vi "inputRead.vi"() -> (10 "ADIO":bool[](array[boolean]), 11 "BDI1":bool[](array[boolean]), 12 "ADI1":bool[](array[boolean]), 13 "BDI0":bool[](array[boolean]), 14 "ADI2":bool[](array[boolean]), 15 "ADI15":bool[](array[boolean]), 16 "ADI3":bool[](array[boolean]), 17 "ADI14":bool[](array[boolean]), 18 "ADI4":bool[](array[boolean]), 19 "ADI13":bool[](array[boolean]), 20 "ADI5":bool[](array[boolean]), 21 "ADI6":bool[](array[boolean]), 22 "ADI7":bool[](array[boolean]), 23 "ADI8":bool[](array[boolean]), 24 "ADI9":bool[](array[boolean]), 25 "ADI10":bool[](array[boolean]), 26 "ADI11":bool[](array[boolean]), 27 "ADI12":bool[](array[boolean]))   [LabVIEW 2019]
uses:
  <vilib>/myRIO/Instrument Drivers/Onboard IO/DIO/typedefs/DIO Reference.ctl
  <vilib>/myRIO/Common/Instrument Driver Framework/Utilities/typedefs/myRIO Generic Hardware Reference.ctl
  <vilib>/myRIO/Common/Instrument Driver Framework/Utilities/typedefs/Hardware Version Enum.ctl
  <vilib>/myRIO/Common/Instrument Driver Framework/Utilities/typedefs/myRIO v1.0 Reference.ctl
  <vilib>/myRIO/Common/Instrument Driver Framework/Utilities/typedefs/Generic FPGA Reference.ctl
  <vilib>/myRIO/Common/Instrument Driver Framework/myRIO v1.0/DIO/typedefs/DIO Channels List.ctl
  <vilib>/myRIO/Common/Instrument Driver Framework/myRIO v1.0/DIO/typedefs/DIO Channels Enum.ctl
  <vilib>/userDefined/High Color/nirio_resource_hc.ctl
  <vilib>/myRIO/Common/Instrument Driver Framework/myRIO v1.0/DIO/vis/myRIO v1.1 Open DIO.vi
  <vilib>/myRIO/Common/Instrument Driver Framework/Utilities/vis/Validate Channels.vi
  <vilib>/myRIO/Common/Instrument Driver Framework/myRIO v1.0/DIO/vis/myRIO v1.0 Reserve DIO.vi
  <vilib>/myRIO/Common/Instrument Driver Framework/myRIO v1.0/DIO/vis/myRIO v1.0 Close DIO.vi
  <vilib>/myRIO/Common/Instrument Driver Framework/myRIO v1.0/Resource Manager/vis/myRIO v1.0 Reserve Channel List.vi
  <vilib>/myRIO/Common/Instrument Driver Framework/myRIO v1.0/DIO/vis/myRIO v1.0 Build MUX Configuration DIO.vi
  <vilib>/myRIO/Common/Instrument Driver Framework/myRIO v1.0/DIO/vis/myRIO v1.0 Unreserve DIO.vi
  <vilib>/myRIO/Common/Instrument Driver Framework/myRIO v1.0/Resource Manager/vis/myRIO v1.0 Reserve Channel.vi
  <vilib>/myRIO/Common/Instrument Driver Framework/myRIO v1.0/Resource Manager/vis/myRIO v1.0 Unreserve Channel.vi
  <vilib>/myRIO/Common/Instrument Driver Framework/myRIO v1.0/Resource Manager/vis/myRIO v1.0 Create Configuration List.vi
  <vilib>/myRIO/Common/Instrument Driver Framework/myRIO v1.0/Resource Manager/vis/myRIO v1.0 Unreserve Channel List.vi
  <vilib>/myRIO/Common/Instrument Driver Framework/myRIO v1.0/Resource Manager/vis/myRIO v1.0 Build Mutex Name.vi
  <vilib>/Utility/VariantDataType/GetNumericInfo.vi
  <vilib>/Utility/error.llb/Error Cluster From Error Code.vi
  <vilib>/myRIO/Common/Instrument Driver Framework/myRIO v1.0/myRIO v1.1 Open.vi
  <vilib>/myRIO/Common/Instrument Driver Framework/Utilities/vis/IO Manager.vi
  <vilib>/myRIO/Common/Instrument Driver Framework/Utilities/vis/Configuration Manager.vi
  <vilib>/myRIO/Common/Instrument Driver Framework/myRIO v1.0/Resource Manager/vis/myRIO v1.0 Configure IO.vi
  <vilib>/myRIO/Common/Instrument Driver Framework/myRIO v1.0/myRIO v1.0 Close.vi
  <vilib>/myRIO/Common/Instrument Driver Framework/myRIO v1.0/DIO/vis/myRIO v1.0 Read DIO.vi
  <vilib>/myRIO/Common/Instrument Driver Framework/myRIO v1.0/DIO/vis/myRIO v1.0 Shutdown DIO.vi
  <vilib>/myRIO/Instrument Drivers/Onboard IO/DIO/vis/myRIO DIO Open.xnode
  <vilib>/myRIO/Instrument Drivers/Onboard IO/DIO/DIO.lvlib
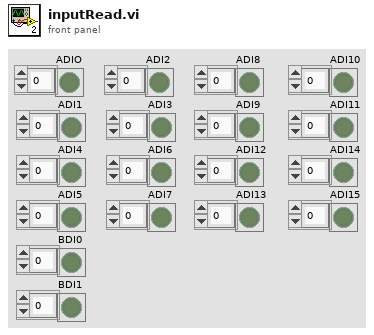
[diagram p1: front panel]
types:
  T1 = typedef "DIO.lvlib/DIO Reference.ctl" = cluster{"myRIO Reference":T2, "DIO Channels List":T6}
  T2 = typedef "myRIO Generic Hardware Reference.ctl" = cluster{"myRIO Model":T3, "myRIO Hardware Reference":T4}
  T3 = typedef "Hardware Version Enum.ctl" = enum16{"Unknown", "myRIO-1900", "myRIO-1950", "roboRIO", "NI ELVIS RIO CM", "ELVIS III"}
  T4 = typedef "myRIO v1.0 Reference.ctl" = cluster{"Generic FPGA Reference":T5, "Allow multiple opens":bool}
  T5 = typedef "Generic FPGA Reference.ctl" = refnum<k20>
  T6 = typedef "DIO Channels List.ctl" = T7[]
  T7 = typedef "DIO Channels Enum.ctl" = enum16{"Not Connected", "C/DIO0", "C/DIO1", "C/DIO2", "C/DIO3", "C/DIO4", "C/DIO5", "C/DIO6", "C/DIO7", "A/DIO0", "A/DIO1", "A/DIO2", "A/DIO3", "A/DIO4", "A/DIO5", "A/DIO6", "A/DIO7", "A/DIO8", "A/DIO9", "A/DIO10", "A/DIO11", "A/DIO12", "A/DIO13", "A/DIO14", "A/DIO15", "A/DIO16", "A/DIO17", "A/DIO18", "A/DIO19", "B/DIO0", "B/DIO1", "B/DIO2", "B/DIO3", "B/DIO4", "B/DIO5", "B/DIO6", "B/DIO7", "B/DIO8", "B/DIO9", "B/DIO10", "B/DIO11", "B/DIO12", "B/DIO13", "B/DIO14", "B/DIO15", "B/DIO16", "B/DIO17", "B/DIO18", "B/DIO19", "LED0", "LED1", "LED2", "LED3", "Button0", "DIO/DIO0", "DIO/DIO1", "DIO/DIO2", "DIO/DIO3", "DIO/DIO4", "DIO/DIO5", "DIO/DIO6", "DIO/DIO7", "DIO/DIO8", "DIO/DIO9", "SPI/CS0", "SPI/CS1", "SPI/CS2", "SPI/CS3", "LED RADIO (Green)", "LED RADIO (Red)", "LED COMM (Green)", "LED COMM (Red)", "LED MODE (Green)", "LED MODE (Red)"}
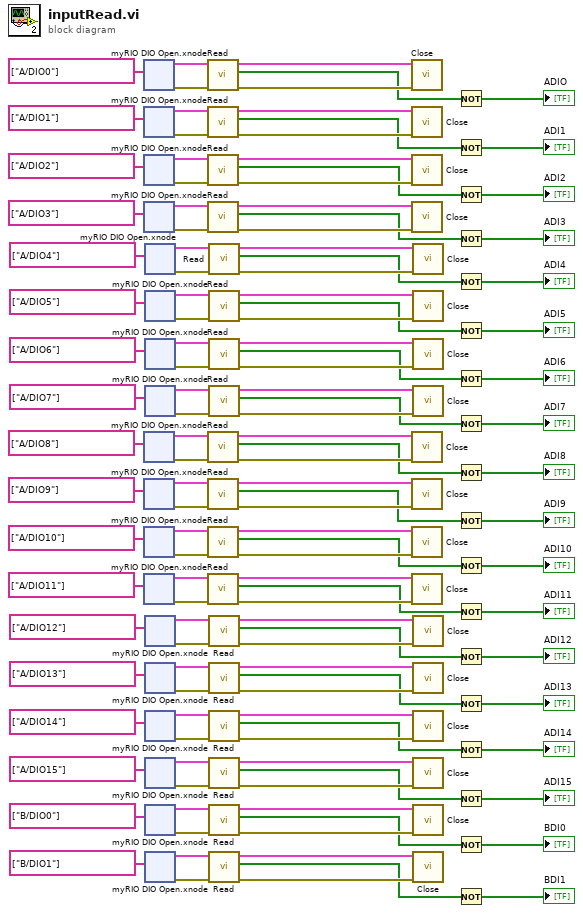
[diagram p0: block diagram]
diagram:
  n1 = xnode "myRIO DIO Open.xnode"("Channel Names"=tag[] ["A/DIO0"]) -> ("error out"=w125:errorcluster, "DIO Ref Out"=w126:T1)  [unwired: 2 in]
  n2 = xnode "myRIO DIO Open.xnode"("Channel Names"=tag[] ["A/DIO1"]) -> ("error out"=w120:errorcluster, "DIO Ref Out"=w121:T1)  [unwired: 2 in]
  n3 = xnode "myRIO DIO Open.xnode"("Channel Names"=tag[] ["A/DIO2"]) -> ("error out"=w115:errorcluster, "DIO Ref Out"=w116:T1)  [unwired: 2 in]
  n4 = xnode "myRIO DIO Open.xnode"("Channel Names"=tag[] ["A/DIO3"]) -> ("error out"=w110:errorcluster, "DIO Ref Out"=w111:T1)  [unwired: 2 in]
  n5 = xnode "myRIO DIO Open.xnode"("Channel Names"=tag[] ["A/DIO8"]) -> ("error out"=w85:errorcluster, "DIO Ref Out"=w86:T1)  [unwired: 2 in]
  n6 = xnode "myRIO DIO Open.xnode"("Channel Names"=tag[] ["A/DIO9"]) -> ("error out"=w80:errorcluster, "DIO Ref Out"=w81:T1)  [unwired: 2 in]
  n7 = xnode "myRIO DIO Open.xnode"("Channel Names"=tag[] ["A/DIO10"]) -> ("error out"=w75:errorcluster, "DIO Ref Out"=w76:T1)  [unwired: 2 in]
  n8 = xnode "myRIO DIO Open.xnode"("Channel Names"=tag[] ["A/DIO11"]) -> ("error out"=w70:errorcluster, "DIO Ref Out"=w71:T1)  [unwired: 2 in]
  n9 = xnode "myRIO DIO Open.xnode"("Channel Names"=tag[] ["A/DIO4"]) -> ("error out"=w105:errorcluster, "DIO Ref Out"=w106:T1)  [unwired: 2 in]
  n10 = xnode "myRIO DIO Open.xnode"("Channel Names"=tag[] ["A/DIO5"]) -> ("error out"=w100:errorcluster, "DIO Ref Out"=w101:T1)  [unwired: 2 in]
  n11 = xnode "myRIO DIO Open.xnode"("Channel Names"=tag[] ["A/DIO6"]) -> ("error out"=w95:errorcluster, "DIO Ref Out"=w96:T1)  [unwired: 2 in]
  n12 = xnode "myRIO DIO Open.xnode"("Channel Names"=tag[] ["A/DIO7"]) -> ("error out"=w90:errorcluster, "DIO Ref Out"=w91:T1)  [unwired: 2 in]
  n13 = xnode "myRIO DIO Open.xnode"("Channel Names"=tag[] ["A/DIO12"]) -> ("error out"=w65:errorcluster, "DIO Ref Out"=w66:T1)  [unwired: 2 in]
  n14 = xnode "myRIO DIO Open.xnode"("Channel Names"=tag[] ["A/DIO13"]) -> ("error out"=w60:errorcluster, "DIO Ref Out"=w61:T1)  [unwired: 2 in]
  n15 = xnode "myRIO DIO Open.xnode"("Channel Names"=tag[] ["A/DIO14"]) -> ("error out"=w55:errorcluster, "DIO Ref Out"=w56:T1)  [unwired: 2 in]
  n16 = xnode "myRIO DIO Open.xnode"("Channel Names"=tag[] ["A/DIO15"]) -> ("error out"=w50:errorcluster, "DIO Ref Out"=w51:T1)  [unwired: 2 in]
  n17 = xnode "myRIO DIO Open.xnode"("Channel Names"=tag[] ["B/DIO0"]) -> ("error out"=w45:errorcluster, "DIO Ref Out"=w46:T1)  [unwired: 2 in]
  n18 = xnode "myRIO DIO Open.xnode"("Channel Names"=tag[] ["B/DIO1"]) -> ("error out"=w40:errorcluster, "DIO Ref Out"=w41:T1)  [unwired: 2 in]
  n19 = call <vilib>:"Read.vi"("error in (no error)"=w125, "DIO Ref In"=w126) -> ("error out"=w123:errorcluster, "Values"=w36:bool[], "DIO Ref Out"=w124:T1)  [unwired: 7 in]
  n20 = call <vilib>:"Read.vi"("error in (no error)"=w120, "DIO Ref In"=w121) -> ("error out"=w118:errorcluster, "Values"=w34:bool[], "DIO Ref Out"=w119:T1)  [unwired: 7 in]
  n21 = call <vilib>:"Read.vi"("error in (no error)"=w115, "DIO Ref In"=w116) -> ("error out"=w113:errorcluster, "Values"=w32:bool[], "DIO Ref Out"=w114:T1)  [unwired: 7 in]
  n22 = call <vilib>:"Read.vi"("error in (no error)"=w110, "DIO Ref In"=w111) -> ("error out"=w108:errorcluster, "Values"=w30:bool[], "DIO Ref Out"=w109:T1)  [unwired: 7 in]
  n23 = call <vilib>:"Read.vi"("error in (no error)"=w85, "DIO Ref In"=w86) -> ("error out"=w83:errorcluster, "Values"=w20:bool[], "DIO Ref Out"=w84:T1)  [unwired: 7 in]
  n24 = call <vilib>:"Read.vi"("error in (no error)"=w80, "DIO Ref In"=w81) -> ("error out"=w78:errorcluster, "Values"=w18:bool[], "DIO Ref Out"=w79:T1)  [unwired: 7 in]
  n25 = call <vilib>:"Read.vi"("error in (no error)"=w75, "DIO Ref In"=w76) -> ("error out"=w73:errorcluster, "Values"=w16:bool[], "DIO Ref Out"=w74:T1)  [unwired: 7 in]
  n26 = call <vilib>:"Read.vi"("error in (no error)"=w70, "DIO Ref In"=w71) -> ("error out"=w68:errorcluster, "Values"=w14:bool[], "DIO Ref Out"=w69:T1)  [unwired: 7 in]
  n27 = call <vilib>:"Read.vi"("error in (no error)"=w105, "DIO Ref In"=w106) -> ("error out"=w103:errorcluster, "Values"=w28:bool[], "DIO Ref Out"=w104:T1)  [unwired: 7 in]
  n28 = call <vilib>:"Read.vi"("error in (no error)"=w100, "DIO Ref In"=w101) -> ("error out"=w98:errorcluster, "Values"=w26:bool[], "DIO Ref Out"=w99:T1)  [unwired: 7 in]
  n29 = call <vilib>:"Read.vi"("error in (no error)"=w95, "DIO Ref In"=w96) -> ("error out"=w93:errorcluster, "Values"=w24:bool[], "DIO Ref Out"=w94:T1)  [unwired: 7 in]
  n30 = call <vilib>:"Read.vi"("error in (no error)"=w90, "DIO Ref In"=w91) -> ("error out"=w88:errorcluster, "Values"=w22:bool[], "DIO Ref Out"=w89:T1)  [unwired: 7 in]
  n31 = call <vilib>:"Read.vi"("error in (no error)"=w65, "DIO Ref In"=w66) -> ("error out"=w63:errorcluster, "Values"=w12:bool[], "DIO Ref Out"=w64:T1)  [unwired: 7 in]
  n32 = call <vilib>:"Read.vi"("error in (no error)"=w60, "DIO Ref In"=w61) -> ("error out"=w58:errorcluster, "Values"=w10:bool[], "DIO Ref Out"=w59:T1)  [unwired: 7 in]
  n33 = call <vilib>:"Read.vi"("error in (no error)"=w55, "DIO Ref In"=w56) -> ("error out"=w53:errorcluster, "Values"=w8:bool[], "DIO Ref Out"=w54:T1)  [unwired: 7 in]
  n34 = call <vilib>:"Read.vi"("error in (no error)"=w50, "DIO Ref In"=w51) -> ("error out"=w48:errorcluster, "Values"=w6:bool[], "DIO Ref Out"=w49:T1)  [unwired: 7 in]
  n35 = call <vilib>:"Read.vi"("error in (no error)"=w45, "DIO Ref In"=w46) -> ("error out"=w43:errorcluster, "Values"=w4:bool[], "DIO Ref Out"=w44:T1)  [unwired: 7 in]
  n36 = call <vilib>:"Read.vi"("error in (no error)"=w40, "DIO Ref In"=w41) -> ("error out"=w38:errorcluster, "Values"=w2:bool[], "DIO Ref Out"=w39:T1)  [unwired: 7 in]
  n37 = call <vilib>:"Close.vi"("error in (no error)"=w123, "DIO Ref In"=w124) -> ()  [unwired: 9 in, 1 out]
  n38 = call <vilib>:"Close.vi"("error in (no error)"=w118, "DIO Ref In"=w119) -> ()  [unwired: 9 in, 1 out]
  n39 = call <vilib>:"Close.vi"("error in (no error)"=w113, "DIO Ref In"=w114) -> ()  [unwired: 9 in, 1 out]
  n40 = call <vilib>:"Close.vi"("error in (no error)"=w108, "DIO Ref In"=w109) -> ()  [unwired: 9 in, 1 out]
  n41 = call <vilib>:"Close.vi"("error in (no error)"=w83, "DIO Ref In"=w84) -> ()  [unwired: 9 in, 1 out]
  n42 = call <vilib>:"Close.vi"("error in (no error)"=w78, "DIO Ref In"=w79) -> ()  [unwired: 9 in, 1 out]
  n43 = call <vilib>:"Close.vi"("error in (no error)"=w73, "DIO Ref In"=w74) -> ()  [unwired: 9 in, 1 out]
  n44 = call <vilib>:"Close.vi"("error in (no error)"=w68, "DIO Ref In"=w69) -> ()  [unwired: 9 in, 1 out]
  n45 = call <vilib>:"Close.vi"("error in (no error)"=w103, "DIO Ref In"=w104) -> ()  [unwired: 9 in, 1 out]
  n46 = call <vilib>:"Close.vi"("error in (no error)"=w98, "DIO Ref In"=w99) -> ()  [unwired: 9 in, 1 out]
  n47 = call <vilib>:"Close.vi"("error in (no error)"=w93, "DIO Ref In"=w94) -> ()  [unwired: 9 in, 1 out]
  n48 = call <vilib>:"Close.vi"("error in (no error)"=w88, "DIO Ref In"=w89) -> ()  [unwired: 9 in, 1 out]
  n49 = call <vilib>:"Close.vi"("error in (no error)"=w63, "DIO Ref In"=w64) -> ()  [unwired: 9 in, 1 out]
  n50 = call <vilib>:"Close.vi"("error in (no error)"=w58, "DIO Ref In"=w59) -> ()  [unwired: 9 in, 1 out]
  n51 = call <vilib>:"Close.vi"("error in (no error)"=w53, "DIO Ref In"=w54) -> ()  [unwired: 9 in, 1 out]
  n52 = call <vilib>:"Close.vi"("error in (no error)"=w48, "DIO Ref In"=w49) -> ()  [unwired: 9 in, 1 out]
  n53 = call <vilib>:"Close.vi"("error in (no error)"=w43, "DIO Ref In"=w44) -> ()  [unwired: 9 in, 1 out]
  n54 = call <vilib>:"Close.vi"("error in (no error)"=w38, "DIO Ref In"=w39) -> ()  [unwired: 9 in, 1 out]
  n55 = Not(x=w36) -> (.not. x?=→"ADIO":bool[])
  n56 = Not(x=w34) -> (.not. x?=→"ADI1":bool[])
  n57 = Not(x=w32) -> (.not. x?=→"ADI2":bool[])
  n58 = Not(x=w30) -> (.not. x?=→"ADI3":bool[])
  n59 = Not(x=w28) -> (.not. x?=→"ADI4":bool[])
  n60 = Not(x=w26) -> (.not. x?=→"ADI5":bool[])
  n61 = Not(x=w24) -> (.not. x?=→"ADI6":bool[])
  n62 = Not(x=w22) -> (.not. x?=→"ADI7":bool[])
  n63 = Not(x=w20) -> (.not. x?=→"ADI8":bool[])
  n64 = Not(x=w18) -> (.not. x?=→"ADI9":bool[])
  n65 = Not(x=w16) -> (.not. x?=→"ADI10":bool[])
  n66 = Not(x=w14) -> (.not. x?=→"ADI11":bool[])
  n67 = Not(x=w12) -> (.not. x?=→"ADI12":bool[])
  n68 = Not(x=w10) -> (.not. x?=→"ADI13":bool[])
  n69 = Not(x=w8) -> (.not. x?=→"ADI14":bool[])
  n70 = Not(x=w6) -> (.not. x?=→"ADI15":bool[])
  n71 = Not(x=w4) -> (.not. x?=→"BDI0":bool[])
  n72 = Not(x=w2) -> (.not. x?=→"BDI1":bool[])
